vi "time jitter.vi"(6 "n":i32=10, 7 "reset":bool, 11 "time (ns)":i64) -> (2 "jitter":dbl, 3 "mean period":dbl)   [LabVIEW 2013]
uses:
  <vilib>/Analysis/NI_AALBase.lvlib
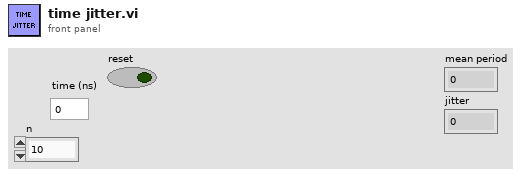
[diagram p1: front panel]
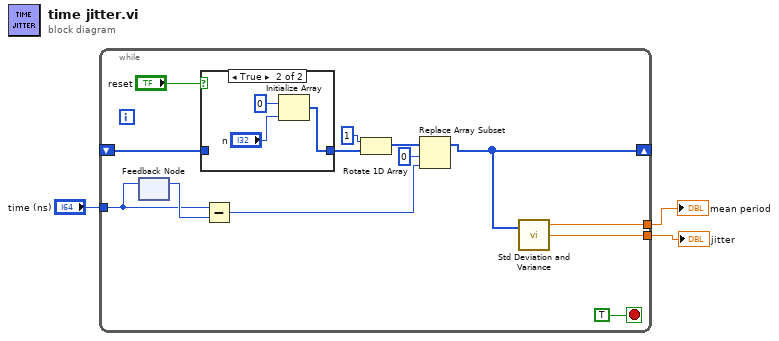
[diagram p0: block diagram]
diagram:
  n1 = while {
    shift-right: [w7] -> _
    shift-left: _ -> [w13]
    tunnel: "time (ns)" -> [w9]
    tunnel: [w6] -> w2
    tunnel: [w5] -> w1
    stop <- TRUE stop-if-true
    n2 = feedback-in #1(w9) -> ()
    n3 = feedback #1() -> (w10:i64)  [unwired: 1 in]
    n4 = case shown="True" "reset" {
      tunnel: [w17 w18] -> w12
      tunnel: w13 -> [w17 _]
      frame False {
      }
      frame True {
        n5 = Initialize Array(i64 0 ("time (ns)"), "n") -> (w18:i64[])
      }
    }
    n6 = Subtract(x=w9, y=w10) -> (x-y=w8:i64)
    n7 = Rotate 1D Array(1:w12, 2:1 ("n")) -> (0:w15:i64[])
    n8 = Replace Array Subset(array=w15, new element=w8, index=0) -> (w7:i64[])
    n9 = call <vilib>:"Std Deviation and Variance.vi"("X"=w7) -> ("mean"=w6:dbl, "standard deviation"=w5:dbl)  [unwired: 1 in, 1 out]
  }
  "mean period" <- w2
  "jitter" <- w1
